vi "Annotate April.vi"(6 "hilight":bool, 7 "Annotate":bool, 9 "cutoffs":T1, 10 "Detected Tags":T3(array[cluster]), 11 "Refnum in":T2) -> (1 "margins":dbl[](array[numeric]), 2 "tags":T3(array[cluster]), 3 "Refnum out":T2)   [LabVIEW 2025]
uses:
  <vilib>/vision/Image Controls.llb/IMAQ Image.ctl
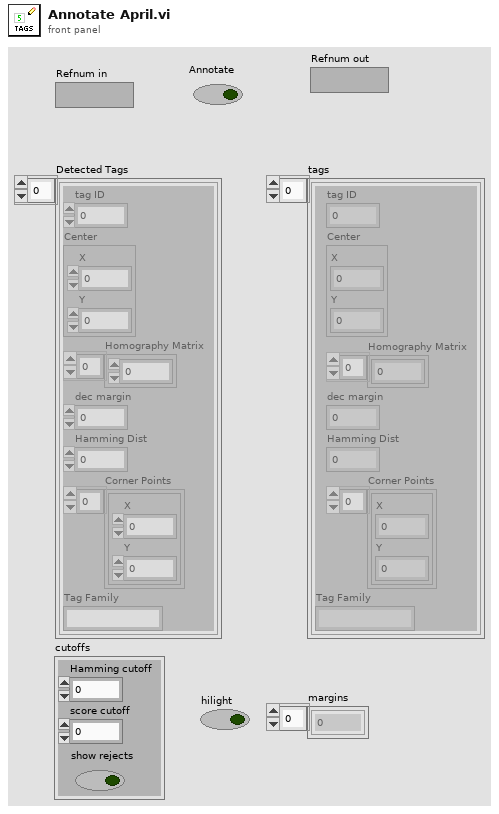
[diagram p1: front panel]
types:
  T1 = cluster{"Hamming cutoff":i32, "score cutoff":dbl, "show rejects":bool}
  T2 = typedef "IMAQ Image.ctl" = refnum<image>
  T3 = cluster{"tag ID":i32, "Center":cluster{"X":dbl, "Y":dbl}, "Homography Matrix":dbl[], "dec margin":dbl, "Hamming Dist":i32, "Corner Points":cluster{"X":dbl, "Y":dbl}[], "Tag Family":string}[]
  T4 = cluster{"Desired Font (Application)":enum16{"User-specified Font", "Application Font", "System Font", "Dialog Font"}, "[User-specified Font]":cluster{"Font Name":string, "Size":i16, "Strikeout?":bool, "Italic?":bool, "Underline?":bool, "Outline?":bool, "Shadow?":bool, "Bold?":bool, "Rotation Angle":dbl}, "Horizontal Alignment":i16, "Vertical Alignment":i16}
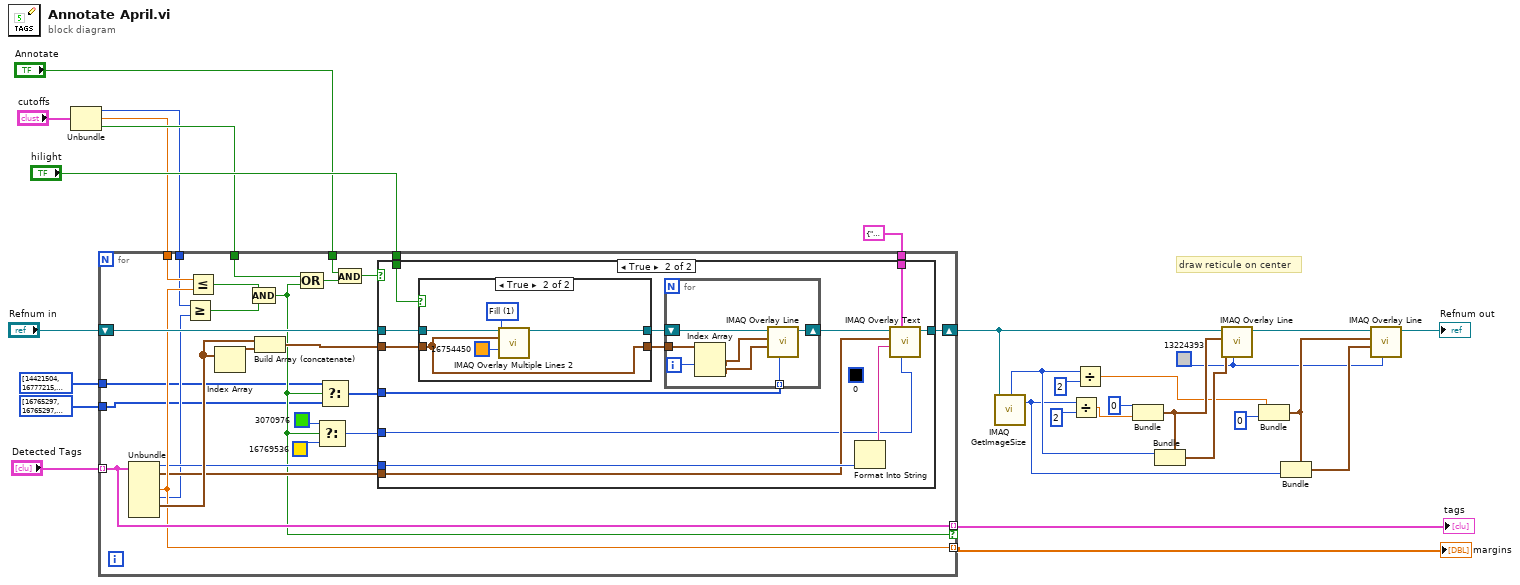
[diagram p0: block diagram]
diagram:
  w10 = u32 13224393 ("Color")
  # "draw reticule on center"
  n1 = Unbundle("cutoffs") -> ("Hamming cutoff"=w4:i32, "score cutoff"=w5:dbl, "show rejects"=w6:bool)
  n2 = for {
    tunnel: "Detected Tags" -> [w53] mode=indexing
    shift-right: [w55] -> w23
    shift-left: "Refnum in" -> [w56]
    tunnel: [w53] -> w29 mode=indexing if=w34
    tunnel: [w52] -> w27 mode=indexing
    tunnel: w6 -> [w44]
    tunnel: T4 {"Desired Font (Application)"=enum."Application Font", "[User-specified Font]"={"Font Name"="", "Size"=12, "Strikeout?"=FALSE, "Italic?"=FALSE, "Underline?"=FALSE, "Outline?"=FALSE, "Shadow?"=FALSE, "Bold?"=FALSE, "Rotation Angle"=0.0}, "Horizontal Alignment"=1, "Vertical Alignment"=2} ("Font, Size & Style") -> [w41]
    tunnel: "hilight" -> [w40]
    tunnel: w5 -> [w39]
    tunnel: w4 -> [w37]
    tunnel: u32[] [14421504, 16777215, 16777215, 3070976] -> [w33]
    tunnel: u32[] [16765297, 16765297, 16765297, 16765297] -> [w32]
    tunnel: "Annotate" -> [w30]
    n3 = Unbundle(w53) -> ("tag ID"=w51:i32, "Center"=w50:cluster{"X":dbl, "Y":dbl}, "dec margin"=w52:dbl, "Hamming Dist"=w38:i32, "Corner Points"=w54:cluster{"X":dbl, "Y":dbl}[])  [unwired: 2 out]
    n4 = Greater Or Equal?(x=w37, y=w38) -> (x >= y?=w35:bool)
    n5 = Less Or Equal?(x=w39, y=w52) -> (x <= y?=w36:bool)
    n6 = Index Array(array=w54) -> (element=w46:cluster{"X":dbl, "Y":dbl})  [unwired: 1 in]
    n7 = Compound Arithmetic op=AND(w36, w35) -> (w34:bool)
    n8 = Build Array (concatenate)(w54, w46) -> (w45:cluster{"X":dbl, "Y":dbl}[])
    n9 = Compound Arithmetic op=OR(w44, w34) -> (w43:bool)
    n10 = Select(t=u32 3070976 ("Color"), s=w34, f=u32 16769536 ("Color")) -> (s? t:f=w47:u32)
    n11 = Select(t=w33, s=w34, f=w32) -> (s? t:f=w42:u32[])
    n12 = And(x=w30, y=w43) -> (x .and. y?=w31:bool)
    n13 = case shown="True" w31 {
      tunnel: w56 -> [w57 w61]
      tunnel: [w57 w70] -> w55
      tunnel: w51 -> [_ w69]
      tunnel: w50 -> [_ w68]
      tunnel: w47 -> [_ w64]
      tunnel: w45 -> [_ w62]
      tunnel: w42 -> [_ w66]
      tunnel: w41 -> [_ w65]
      tunnel: w40 -> [_ w58]
      frame False {
      }
      frame True {
        (unwired) u32 0 ("Color")
        n14 = case shown="True" w58 {
          tunnel: w62 -> [w71 w74]
          tunnel: w61 -> [w72 w76]
          tunnel: [w72 w77] -> w60
          tunnel: [w71 w74] -> w59
          frame False {
          }
          frame True {
            w73 = u32 1 items=["Frame", "Fill"] ("Drawing Mode (Frame)")
            n15 = call "IMAQ Overlay Multiple Lines 2"("Image"=w76, "Line End Points"=w74, "Drawing Mode (Frame)"=w73, "Color"=u32 16754450) -> ("Image Out"=w77:T2)  [unwired: 10 in, 1 out]
          }
        }
        n16 = for {
          shift-right: [w78] -> w63
          shift-left: w60 -> [w84]
          tunnel: w59 -> [w83]
          tunnel: w66 -> [w81] mode=indexing
          i -> [w82]
          n17 = Index Array(array=w83, index #1=w82) -> (element #1=w79:cluster{"X":dbl, "Y":dbl}, element #2=w80:cluster{"X":dbl, "Y":dbl})  [unwired: 1 in]
          n18 = call "IMAQ Overlay Line"("Color"=w81, "End Point"=w80, "Start Point"=w79, "Image"=w84) -> ("Image Out"=w78:T2)  [unwired: 6 in, 1 out]
        }
        n19 = Format Into String(w69) -> (resulting string=w67:string)  [unwired: 3 in, 1 out]
        n20 = call "IMAQ Overlay Text"("Text Color (black)"=w64, "Font, Size & Style"=w65, "String"=w67, "Origin"=w68, "Image"=w63) -> ("Image Out"=w70:T2)  [unwired: 5 in, 1 out]
      }
    }
  }
  "tags" <- w29
  "margins" <- w27
  n21 = call "IMAQ GetImageSize"("Image"=w23) -> ("Y Resolution"=w13:i32, "X Resolution"=w18:i32)  [unwired: 3 in, 1 out]
  n22 = Divide(x=w13, y=2 ("X")) -> (x/y=w20:dbl)
  n23 = Divide(x=w18, y=2 ("X")) -> (x/y=w14:dbl)
  n24 = Bundle("X"=0, w20) -> (w19:cluster{"X":i32, dbl})  [unwired: 1 in]
  n25 = Bundle(cluster=w19, "X"=w18) -> (w17:cluster{"X":i32, dbl})  [unwired: 1 in]
  n26 = call "IMAQ Overlay Line"("Color"=w10, "End Point"=w17, "Start Point"=w19, "Image"=w23) -> ("Image Out"=w25:T2)  [unwired: 6 in, 1 out]
  n27 = Bundle(w14, "X"=0) -> (w11:cluster{dbl, "X":i32})  [unwired: 1 in]
  n28 = Bundle(cluster=w11, "X"=w13) -> (w12:cluster{dbl, "X":i32})  [unwired: 1 in]
  n29 = call "IMAQ Overlay Line"("Color"=w10, "End Point"=w12, "Start Point"=w11, "Image"=w25) -> ("Image Out"=→"Refnum out":T2)  [unwired: 6 in, 1 out]
